vi "Valco Send Command.vi"(8 "error in (no error)":errorcluster, 10 "Command":string, 11 "VISA resource name in":refnum<visa-resource-name>="COM3") -> (0 "error out":errorcluster, 3 "VISA resource name out":refnum<visa-resource-name>)   [LabVIEW 2018]
panel:
  out "Response":string
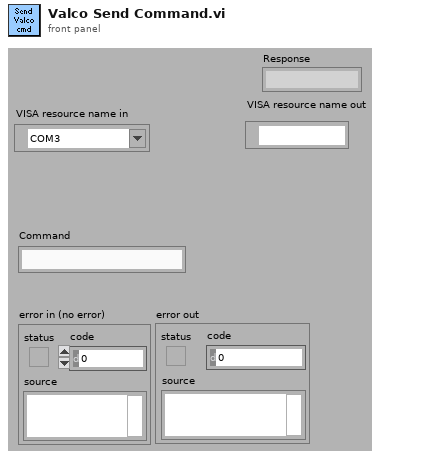
[diagram p1: front panel]
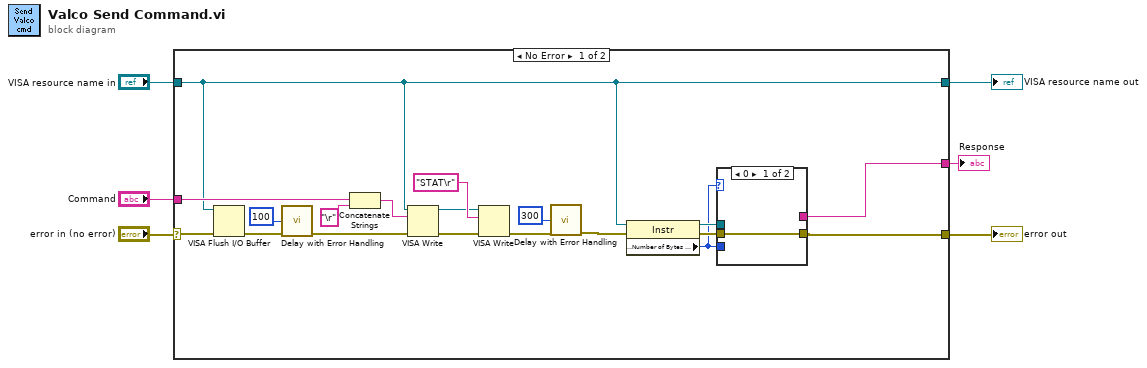
[diagram p0: block diagram]
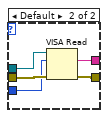
[diagram p2: hidden frame]
diagram:
  n1 = case shown="No Error" "error in (no error)" {
    selector: "error in (no error)" -> [w22 w33]
    tunnel: "Command" -> [w15 _]
    tunnel: [w8 w33] -> w4
    tunnel: "VISA resource name in" -> [w9 w32]
    tunnel: [w9 w32] -> w2
    tunnel: [w7 _] -> w1
    frame No Error {
      n2 = VISA Flush I/O Buffer(VISA resource name=w9, error in (no error)=w22) -> (error out=w21:errorcluster)  [unwired: 1 in, 1 out]
      n3 = call "Delay with Error Handling.vi"("error in (no error)"=w21, "Delay (ms)"=u32 100) -> ("error out"=w14:errorcluster)  [unwired: 9 in]
      n4 = Concatenate Strings(w15, "\r" ("string")) -> (w25:string)
      n5 = VISA Write(VISA resource name=w9, write buffer=w25, error in (no error)=w14) -> (VISA resource name out=w18:refnum<visa-resource-name>, error out=w20:errorcluster)  [unwired: 1 out]
      n6 = VISA Write(VISA resource name=w18, write buffer="STAT\r" ("string"), error in (no error)=w20) -> (error out=w16:errorcluster)  [unwired: 2 out]
      n7 = call "Delay with Error Handling.vi"("error in (no error)"=w16, "Delay (ms)"=u32 300) -> ("error out"=w10:errorcluster)  [unwired: 9 in]
      n8 = property class="Instr"(reference=w9, error in=w10) -> (reference out=w12:refnum<visa-resource-name>, error out=w13:errorcluster, "Serial Settings:Number of Bytes at Serial Port"=w11:u32)
      n9 = case shown="0" w11 {
        tunnel: w13 -> [w26 w31]
        tunnel: w12 -> [_ w30]
        tunnel: w11 -> [_ w29]
        tunnel: [w26 w28] -> w8
        tunnel: [_ w27] -> w7
        frame 0 {
        }
        frame Default {
          n10 = VISA Read(VISA resource name=w30, byte count=w29, error in (no error)=w31) -> (read buffer=w27:string, error out=w28:errorcluster)  [unwired: 2 out]
        }
      }
    }
    frame Error {
    }
  }
  "error out" <- w4
  "VISA resource name out" <- w2
  "Response" <- w1
